vi "Stop All DAQ.vi"(8 "error in (no error)":errorcluster, 10 "final error code":i32, 11 "Cfg Grandmaster in":refnum<class "Cfg Grandmaster.lvclass">) -> (0 "error out":errorcluster, 3 "Cfg Grandmaster out":refnum<class "Cfg Grandmaster.lvclass">)   [LabVIEW 2018, in "Configuration Grandmaster.lvlib" / "Cfg Grandmaster.lvclass"]
uses:
  Cfg Grandmaster.lvclass
  C:/Program Files (x86)/National Instruments/LabVIEW 2018/vi.lib/ActorFramework/Actor/Actor.lvclass
  Cfg Grandmaster.lvclass/Cfg Grandmaster.ctl
  Common/Controls/DAQMan Mode.ctl
  <vilib>/ActorFramework/Actor/Actor.lvclass/Actor.ctl
  <vilib>/ActorFramework/Message Enqueuer/Message Enqueuer.lvclass/Message Enqueuer.ctl
  <vilib>/ActorFramework/Message Enqueuer/Init from Existing Queue.vi
  Cfg Grandmaster Messages/Stop DAQ Timeout Msg/Stop DAQ Timeout Msg.lvclass
  C:/Program Files (x86)/National Instruments/LabVIEW 2018/vi.lib/ActorFramework/Message/Message.lvclass
  <vilib>/ActorFramework/Message Enqueuer/Message Enqueuer.lvclass
  Data Acquisition/Class Chassis Tasks/Chassis Tasks.lvclass
  Class FP Ctrls/FP Controls.lvclass
  <vilib>/ActorFramework/Actor/Actor.lvclass
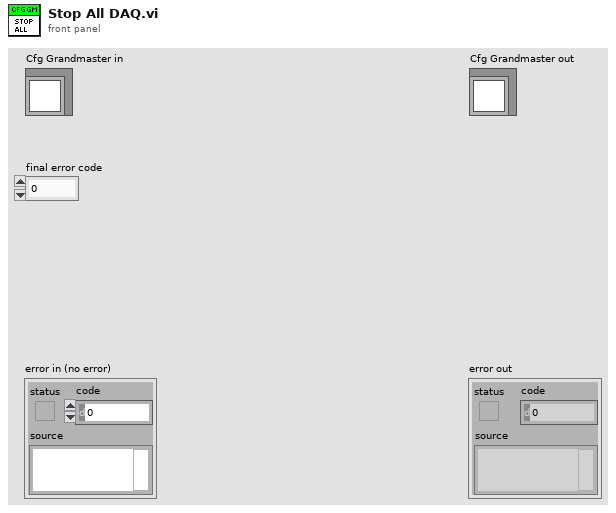
[diagram p1: front panel]
types:
  T1 = typedef "DAQMan Mode.ctl" = enum16{"Cfg", "Run", "Shutting Down"}
  T2 = typedef "ge_Cfg wChassis.ctl" = cluster{"Chassis BOM":refnum<class "Chassis BOM.lvclass">, "Chassis Cfg":refnum<class "ChassisCfg.lvclass">, "Chassis Tasks":refnum<class "Chassis Tasks.lvclass">, "HW Error":bool, "Unsvd Chgs?":bool}
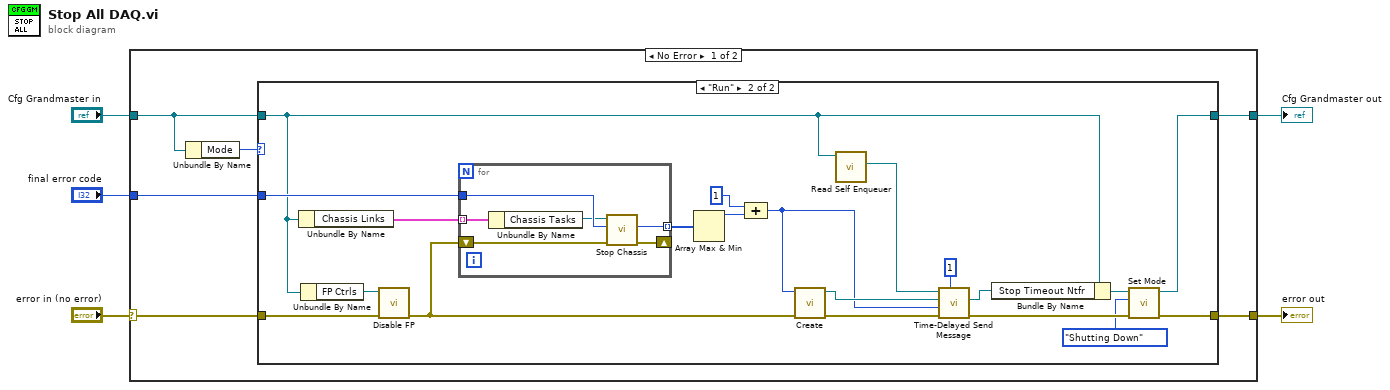
[diagram p0: block diagram]
diagram:
  n1 = case shown="No Error" "error in (no error)" {
    selector: "error in (no error)" -> [w11 w41]
    tunnel: [w9 w41] -> w4
    tunnel: [w8 w40] -> w2
    tunnel: "Cfg Grandmaster in" -> [w7 w40]
    tunnel: "final error code" -> [w10 _]
    frame No Error {
      n2 = Unbundle By Name(w7) -> ("Mode"=w6:T1)
      n3 = case shown="\"Run\"" w6 {
        tunnel: w11 -> [w12 w33]
        tunnel: w10 -> [_ w31]
        tunnel: [w12 w18] -> w9
        tunnel: [w13 w16] -> w8
        tunnel: w7 -> [w13 w20]
        frame Default {
        }
        frame "Run" {
          n4 = Unbundle By Name(w20) -> ("Chassis Links"=w30:T2[])
          n5 = Unbundle By Name(w20) -> ("FP Ctrls"=w32:refnum<class "FP Controls.lvclass">)
          n6 = call "Disable FP.vi"("error in (no error)"=w33, "FP Controls in"=w32) -> ("error out"=w28:errorcluster)  [unwired: 8 in, 1 out]
          n7 = for {
            tunnel: w30 -> [w39] mode=indexing
            tunnel: w31 -> [w37]
            shift-right: [w38] -> _
            shift-left: w28 -> [w35]
            tunnel: [w34] -> w29 mode=indexing
            n8 = Unbundle By Name(w39) -> ("Chassis Tasks"=w36:refnum<class "Chassis Tasks.lvclass">)
            n9 = call-dynamic "Stop Chassis.vi"("error in (no error)"=w35, "final error code"=w37, "Chassis Tasks in"=w36) -> ("error out"=w38:errorcluster, "Max Read Time (ms)"=w34:i32)  [unwired: 6 in, 1 out]
          }
          n10 = Array Max & Min(array=w29) -> (max value=w27:i32)  [unwired: 3 out]
          n11 = Compound Arithmetic op=ADD(1 ("value"), w27) -> (w24:i32)
          n12 = call "Create.vi"("error in (no error)"=w28, "Timeout"=w24) -> ("error out"=w26:errorcluster, "Stop DAQ Timeout Msg out"=w25:refnum<class "Stop DAQ Timeout Msg.lvclass">)  [unwired: 8 in]
          n13 = call <vilib>:"Read Self Enqueuer.vi"("Actor"=w20) -> ("Self Enqueuer"=w22:refnum<class "Message Enqueuer.lvclass">)  [unwired: 10 in]
          n14 = call <vilib>:"Time-Delayed Send Message.vi"("# Copies (0 = infinite repeat)"=u32 1, "error in (no error)"=w26, "Milliseconds To Wait"=w24, "Message"=w25, "Message Enqueuer"=w22) -> ("error out"=w19:errorcluster, "Delivery Notifier"=w21:refnum<notifier>)  [unwired: 5 in]
          n15 = Bundle By Name(cluster=w20, "Stop Timeout Ntfr"=w21) -> (w17:refnum<class "Cfg Grandmaster.lvclass">)
          n16 = call "Set Mode.vi"("error in (no error)"=w19, "Mode"=DAQMan_Mode."Shutting Down", "Cfg Grandmaster in"=w17) -> ("error out"=w18:errorcluster, "Cfg Grandmaster out"=w16:refnum<class "Cfg Grandmaster.lvclass">)  [unwired: 7 in]
        }
      }
    }
    frame Error {
    }
  }
  "error out" <- w4
  "Cfg Grandmaster out" <- w2
